vi "Do Something.vi"(8 "error in (no error)":errorcluster, 11 "ByRef Add in":refnum<class "ByRef Add.lvclass">) -> (0 "error out":errorcluster, 3 "ByRef Add out":refnum<class "ByRef Add.lvclass">)   [LabVIEW 2020, in "ByRef Add.lvclass"]
uses:
  ByRef Add.lvclass
  C:/dev/LabVIEW/ByRef & Callbacks/ByRef Base/ByRef Base.lvclass
  ByRef Base/ByRef Base.lvclass
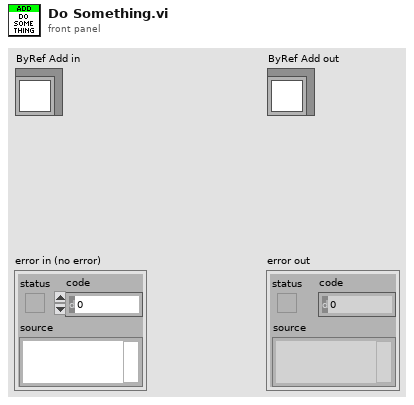
[diagram p1: front panel]
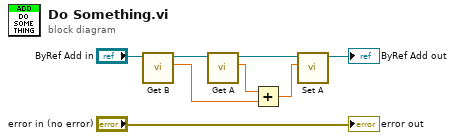
[diagram p0: block diagram]
diagram:
  n1 = call "Get B.vi"("ByRef Base in"="ByRef Add in") -> ("B"=w1:dbl, "ByRef Base out"=w2:refnum<class "ByRef Add.lvclass">)  [unwired: 8 in, 1 out]
  n2 = call "Get A.vi"("ByRef Base in"=w2) -> ("Numeric"=w6:dbl, "ByRef Base out"=w8:refnum<class "ByRef Add.lvclass">)  [unwired: 8 in, 1 out]
  n3 = Add(x=w6, y=w1) -> (x+y=w5:dbl)
  n4 = call "Set A.vi"("Numeric"=w5, "ByRef Base in"=w8) -> ("ByRef Base out"=→"ByRef Add out":refnum<class "ByRef Add.lvclass">)  [unwired: 8 in, 1 out]
  "error out" <- "error in (no error)"
